vi "Becker-Hickl Read Single U32.vi"(8 "Error In":errorcluster, 10 "Default":u32, 11 "Bytes in":string) -> (0 "Error Out":errorcluster, 2 "U32":u32, 3 "Bytes out":string)   [LabVIEW 2021, in "Becker-Hickl Files.lvlib"]
uses:
  Becker-Hickl Files.lvlib
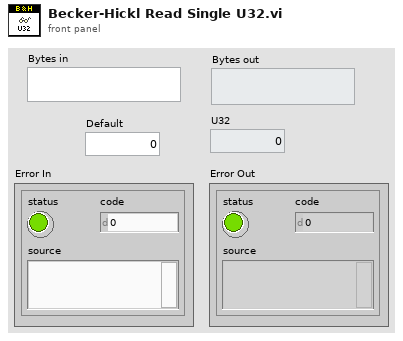
[diagram p1: front panel]
types:
  T1 = enum16{"big-endian, network order", "native, host order", "little-endian"}
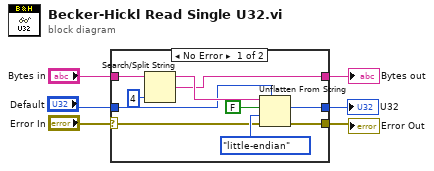
[diagram p0: block diagram]
diagram:
  n1 = case shown="No Error" "Error In" {
    selector: "Error In" -> [w9 w18]
    tunnel: [w16 w17] -> w6
    tunnel: [w12 w19] -> w5
    tunnel: "Bytes in" -> [w15 w19]
    tunnel: [w8 w18] -> w2
    tunnel: "Default" -> [w7 w17]
    frame No Error {
      n2 = Search/Split String(string=w15, offset (0)=4 ("index")) -> (substring before match=w13:string, match + rest of string=w12:string)  [unwired: 1 in, 1 out]
      n3 = Unflatten From String(type=w7, binary string=w13, data includes array or string size? (T)=FALSE, byte order (0:big-endian, network order)=T1."little-endian", error in (no error)=w9) -> (value=w16:u32, error out=w8:errorcluster)  [unwired: 1 out]
    }
    frame Error {
    }
  }
  "U32" <- w6
  "Bytes out" <- w5
  "Error Out" <- w2
